vi "Fit.vi"(8 "error in (no error)":errorcluster caption="entrée d'erreur (pas d'erreur)", 9 "y":string[][](array[string]), 10 "X":string[][](array[string]), 11 "Normalizer.lvclass":refnum<class "Normalizer.lvclass">) -> (0 "error out":errorcluster caption="sortie d'erreur", 2 "String Data":string, 3 "Normalizer.lvclass":refnum<class "Normalizer.lvclass">)   [LabVIEW 2020, in "Normalizer.lvclass"]
doc: "Do nothing and return the estimator unchanged\n\nThis method is just there to implement the usual API and hence work in pipelines.\n\nReturns : \n\n- String : OK"
uses:
  Normalizer.lvclass
  Normalizer.lvclass/Normalizer.ctl
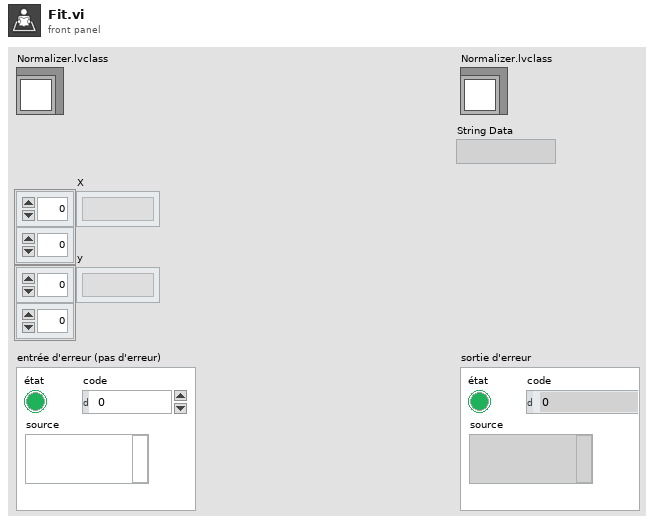
[diagram p1: front panel]
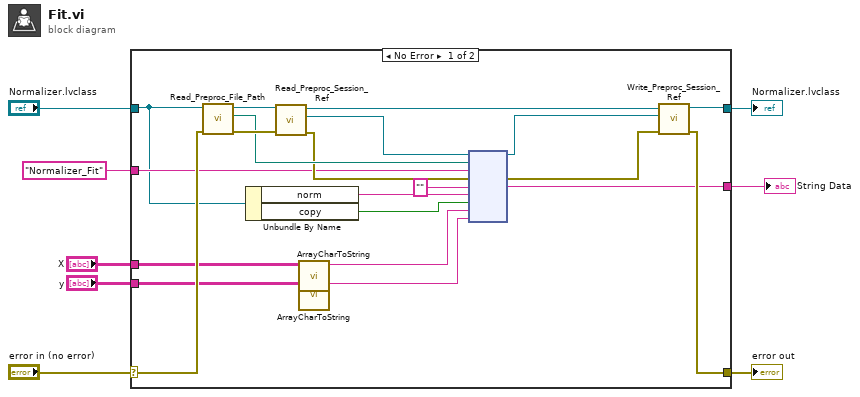
[diagram p0: block diagram]
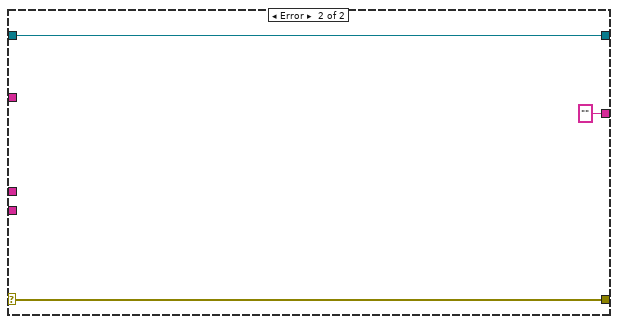
[diagram p2: hidden frame]
diagram:
  n1 = case shown="No Error" "error in (no error)" {
    selector: "error in (no error)" -> [w18 w32]
    tunnel: [w16 w32] -> w7
    tunnel: [w17 w31] -> w5
    tunnel: "Normalizer.lvclass" -> [w13 w31]
    tunnel: "Normalizer_Fit" ("Fonction") -> [w15 _]
    tunnel: [w14 ""] -> w3
    tunnel: "X" -> [w12 _]
    tunnel: "y" -> [w11 _]
    frame No Error {
      n2 = call-dynamic "Read_Preproc_File_Path.vi"("error in (no error)"=w18, "Python in"=w13) -> ("error out"=w28:errorcluster, "File_Path"=w25:path, "Python out"=w29:refnum<class "Normalizer.lvclass">)  [unwired: 7 in]
      n3 = Unbundle By Name(w13) -> ("norm"=w20:string, "copy"=w19:bool)
      n4 = call-dynamic "Read_Preproc_Session_Ref.vi"("error in (no error)"=w28, "Python in"=w29) -> ("error out"=w24:errorcluster, "Session_ref"=w26:refnum<k35>, "Python out"=w27:refnum<class "Normalizer.lvclass">)  [unwired: 7 in]
      n5 = call "ArrayCharToString.vi"("TAB"=w12) -> ("Instruction"=w10:string)  [unwired: 10 in]
      n6 = call "ArrayCharToString.vi"("TAB"=w11) -> ("Instruction"=w9:string)  [unwired: 10 in]
      n7 = node(w26, w25, w15, w24, "", w20, w19, w10, w9) -> (w22:refnum<k35>, w23:errorcluster, w14:string)  [unwired: 4 in, 2 out]
      n8 = call-dynamic "Write_Preproc_Session_Ref.vi"("error in (no error)"=w23, "Session_ref"=w22, "Python in"=w27) -> ("error out"=w16:errorcluster, "Python out"=w17:refnum<class "Normalizer.lvclass">)  [unwired: 7 in]
    }
    frame Error {
    }
  }
  "error out" <- w7
  "Normalizer.lvclass" <- w5
  "String Data" <- w3
